vi "checkReceptorPosition.vi"(6 "target":dbl[](array[numeric]), 7 "Game":refnum<class "Game.lvclass">, 8 "error in (no error)":errorcluster, 9 "role":T1=enum."WaitPass", 10 "OffensiveRobots":refnum<class "Robot.lvclass">[](array[class]), 11 "KickToPassReceiverTactic in":refnum<class "KickToPassReceiverTactic.lvclass">) -> (0 "error out":errorcluster, 1 "finalTarget":dbl[](array[numeric]), 2 "calculateForce":bool, 3 "KickToPassReceiverTactic out":refnum<class "KickToPassReceiverTactic.lvclass">, 5 "distReceiverToBall":dbl)   [LabVIEW 2020, in "KickToPassReceiverTactic.lvclass"]
uses:
  KickToPassReceiverTactic.lvclass
  Robot_class/Robot.lvclass
  C:/RoboIME/SSL_AI/Object_class/Object.lvclass
  Robot_class/roles.ctl
  Game_class/Game.lvclass
  Utilities_class/Utilities.lvclass
  Game_class/Game.lvclass/Game.ctl
  Object_class/Object.lvclass/Object.ctl
  Parameters_class/Parameters.lvclass/Parameters.ctl
  Game_class/Read Parameters.lvclass.vi
  Parameters_class/Read AttakingOurselves.vi
  Game_class/Read FieldRef.vi
  Object_class/Read x.vi
  Object_class/Read y.vi
  Field_class/Field.lvclass
  Parameters_class/Parameters.lvclass
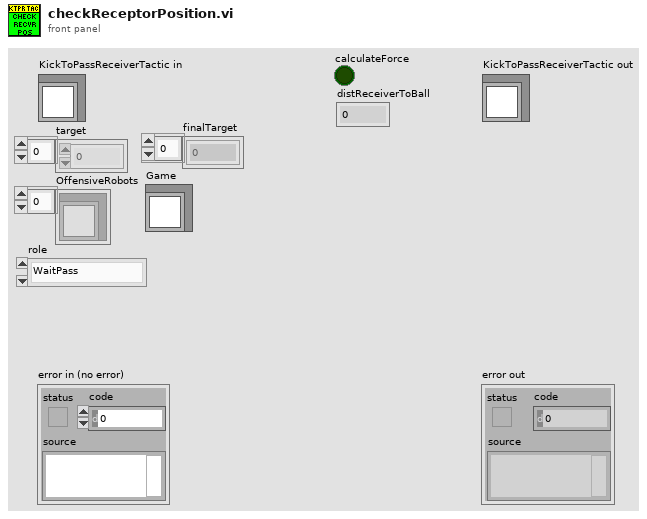
[diagram p1: front panel]
types:
  T1 = typedef "roles.ctl" = enum16{"SecondMarker", "5Robots5th", "PassBestReceiver", "5Robots4th", "5Robots3rd", "5Robots2nd", "5Robots1st", "PassBestRobot", "WaitPass", "ABCThirdKicker", "ABCFirstKicker", "ABCSecondKicker", "Tabler", "TableFinalizer", "PrepareRollToPassRoller", "PrepareRollToPassReceiver", "SimplePassRoll", "SimplePassRollReceiver", "PenaltyDefense", "PreparePassReceiver 2", "PreparePassReceiver 1", "PassObserver", "Timeout", "Goto", "ZigZag", "None", "BallOutOfField", "DefenderArea", "Duelist", "AttackerStop", "FollowAttacker", "KeeperRole", "KickPenalty", "AttackerAimGoal", "AttackerBlock", "Marker", "Halt", "Shoot", "PassKicker", "PassReceiver", "TestRole", "PenaltyAttacker"}
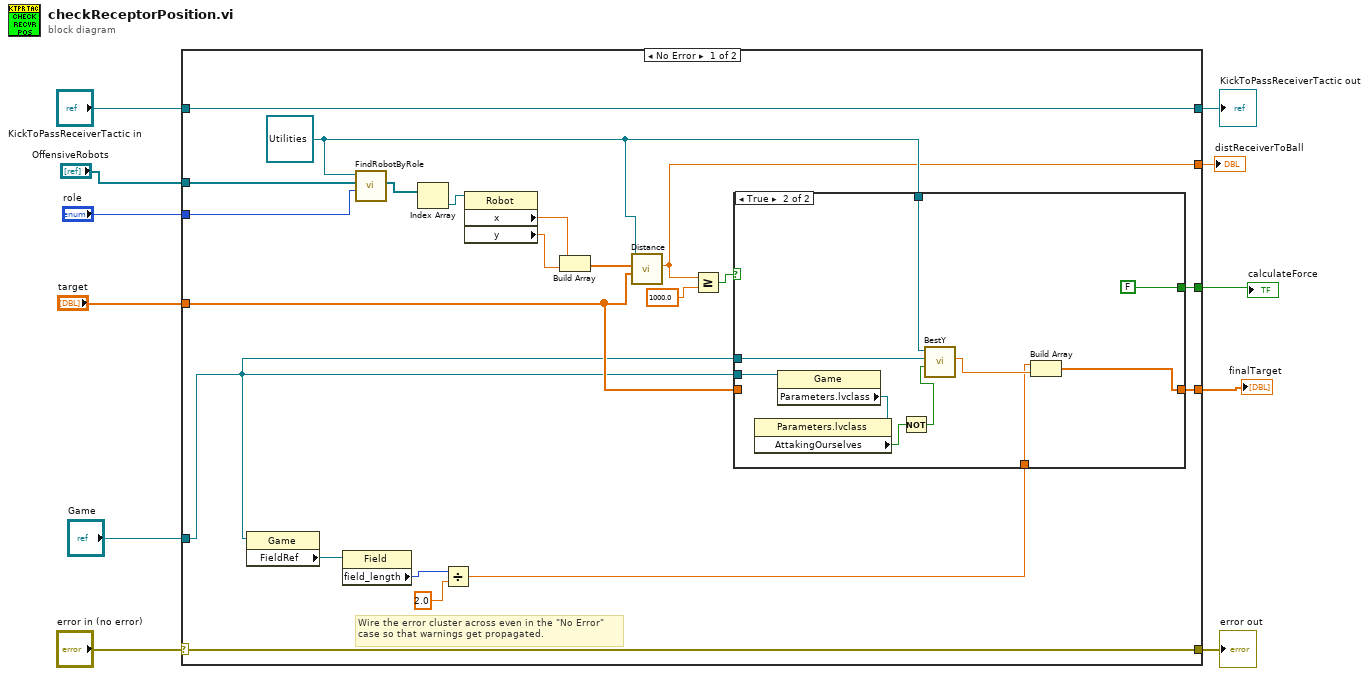
[diagram p0: block diagram]
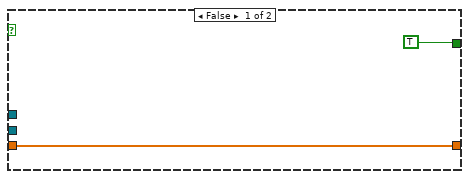
[diagram p2: hidden frame]
diagram:
  n1 = case shown="No Error" "error in (no error)" {
    selector: "error in (no error)" -> [w31 w46]
    tunnel: [w31 w46] -> w10
    tunnel: [w32 w45] -> w8
    tunnel: "KickToPassReceiverTactic in" -> [w32 w45]
    tunnel: "OffensiveRobots" -> [w30 _]
    tunnel: "role" -> [w29 _]
    tunnel: "target" -> [w19 _]
    tunnel: [w21 _] -> w4
    tunnel: [w20 _] -> w3
    tunnel: "Game" -> [w13 _]
    tunnel: [w12 _] -> w1
    frame No Error {
      w15 = refnum<class "Utilities.lvclass"> refnum ("Utilities in")
      # "Wire the error cluster across even in the \"No Error\"\ncase so that warnings get propagated."
      n2 = property class="Game"(reference=w13) -> ("FieldRef"=w18:refnum<class "Field.lvclass">)  [unwired: 1 in, 2 out]
      n3 = property class="Field"(reference=w18) -> ("field_length"=w17:i32)  [unwired: 1 in, 2 out]
      n4 = call "FindRobotByRole.vi"("role"=w29, "RobotRef"=w30, "Utilities in"=w15) -> ("Robots"=w28:refnum<class "Robot.lvclass">[])  [unwired: 6 in, 2 out]
      n5 = Index Array(array=w28) -> (element=w27:refnum<class "Robot.lvclass">)  [unwired: 1 in]
      n6 = Divide(x=w17, y=2.0) -> (x/y=w14:dbl)
      n7 = property class="Robot"(reference=w27) -> ("x"=w26:dbl, "y"=w25:dbl)  [unwired: 1 in, 2 out]
      n8 = Build Array(w26, w25) -> (w22:dbl[])
      n9 = call "Distance.vi"("P1"=w19, "P2"=w22, "Utilities in"=w15) -> ("Distance"=w12:dbl)  [unwired: 6 in, 2 out]
      n10 = Greater Or Equal?(x=w12, y=1000.0) -> (x >= y?=w23:bool)
      n11 = case shown="True" w23 {
        tunnel: [TRUE FALSE] -> w21
        tunnel: [w33 w40] -> w20
        tunnel: w19 -> [w33 _]
        tunnel: w15 -> [_ w43]
        tunnel: w14 -> [_ w41]
        tunnel: w13 -> [_ w39]
        tunnel: w13 -> [_ w36]
        frame False {
        }
        frame True {
          n12 = property class="Game"(reference=w36) -> ("Parameters.lvclass"=w37:refnum<class "Parameters.lvclass">)  [unwired: 1 in, 2 out]
          n13 = property class="Parameters.lvclass"(reference=w37) -> ("AttakingOurselves"=w38:bool)  [unwired: 1 in, 2 out]
          n14 = Not(x=w38) -> (.not. x?=w35:bool)
          n15 = call "BestY.vi"("Utilities in"=w43, "Game"=w39, "inimigos"=w35) -> ("Best y"=w42:dbl)  [unwired: 2 in, 4 out]
          n16 = Build Array(w41, w42) -> (w40:dbl[])
        }
      }
    }
    frame Error {
    }
  }
  "error out" <- w10
  "KickToPassReceiverTactic out" <- w8
  "calculateForce" <- w4
  "finalTarget" <- w3
  "distReceiverToBall" <- w1
